vi "ReturnHome.vi"(8 "Steps/Rev":dbl, 9 "Y Position":dbl, 10 "X Position":dbl, 11 "task in":refnum<k21>) -> (3 "task out":refnum<k21>)   [LabVIEW 2024]
panel:
  in  "Return Home Bool":bool
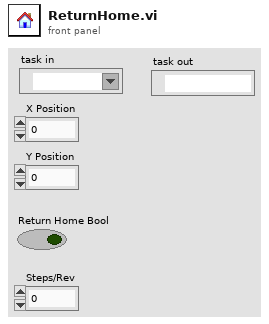
[diagram p1: front panel]
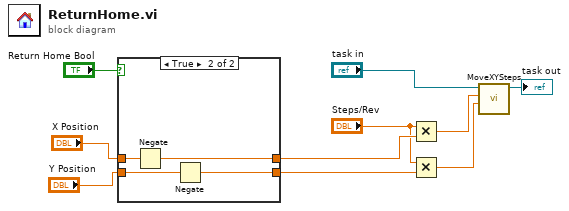
[diagram p0: block diagram]
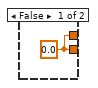
[diagram p2: hidden frame]
diagram:
  n1 = case shown="True" "Return Home Bool" {
    tunnel: "Y Position" -> [_ w15]
    tunnel: "X Position" -> [_ w14]
    tunnel: [w11 w13] -> w4
    tunnel: [w11 w12] -> w5
    frame False {
      w11 = 0.0
    }
    frame True {
      n2 = Negate(x=w14) -> (-x=w12:dbl)
      n3 = Negate(x=w15) -> (-x=w13:dbl)
    }
  }
  n4 = Multiply(x="Steps/Rev", y=w5) -> (x*y=w10:dbl)
  n5 = Multiply(x="Steps/Rev", y=w4) -> (x*y=w9:dbl)
  n6 = call "MoveXYSteps.vi"("Y Steps"=w9, "X Steps"=w10, "task in"="task in") -> ("task out"=→"task out":refnum<k21>)  [unwired: 8 in]
